vi "Data_select.vi"(6 "g(k) in 2":dbl[][](array[numeric]), 7 "s(k) Corregido":dbl[][](array[numeric]), 8 "m":i32=2, 9 "P":i32=64, 10 "s(k) in":dbl[][](array[numeric]), 11 "g(k) in":dbl[][](array[numeric])) -> (0 "s(k) lineal Corregido":ext[](array[numeric]), 1 "s(k) lineal":ext[](array[numeric]), 2 "g(k)lineal_2":ext[](array[numeric]), 3 "g(k) lineal":ext[](array[numeric]))   [LabVIEW 2015]
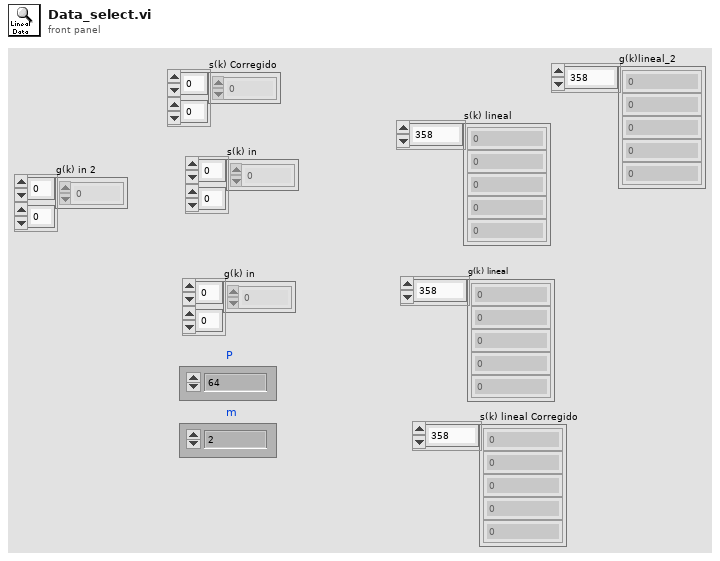
[diagram p1: front panel]
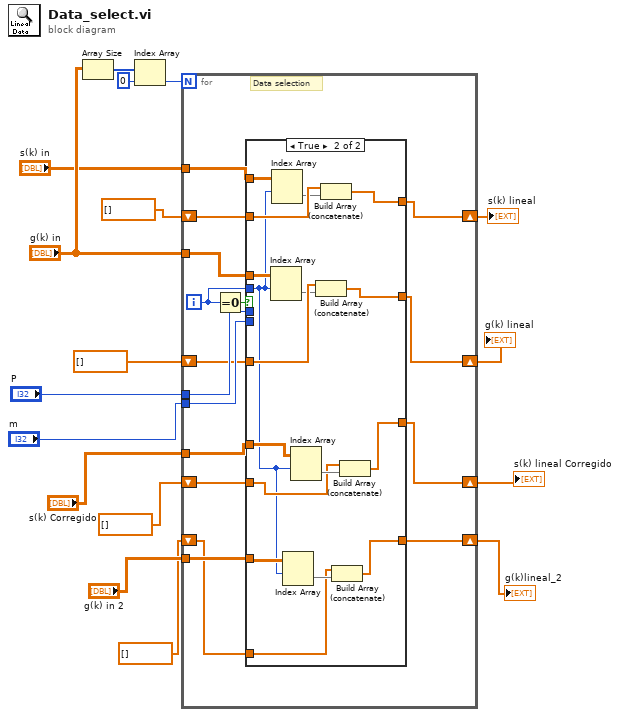
[diagram p0: block diagram]
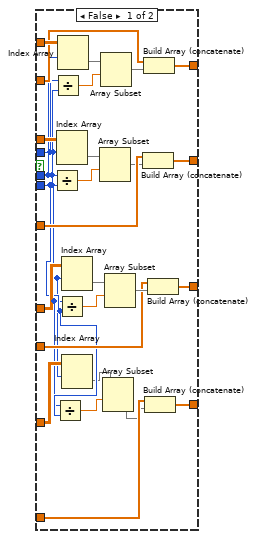
[diagram p2: hidden frame]
diagram:
  n1 = Array Size(array="g(k) in") -> (size(s)=w16:i32[])
  n2 = Index Array(array=w16, index=0) -> (element=w14:i32)
  n3 = for {
    N: w14 -> [_]
    tunnel: "g(k) in" -> [w32]
    tunnel: "m" -> [w30]
    tunnel: "P" -> [w29]
    shift-right: [w27] -> w10
    shift-left: ext[] [] ("Photon trace A") -> [w28]
    tunnel: "s(k) in" -> [w26]
    shift-right: [w24] -> w7
    shift-left: ext[] [] ("Photon trace A") -> [w25]
    tunnel: "s(k) Corregido" -> [w23]
    shift-right: [w21] -> w4
    shift-left: ext[] [] ("Photon trace A") -> [w22]
    tunnel: "g(k) in 2" -> [w20]
    shift-right: [w18] -> w1
    shift-left: ext[] [] ("Photon trace A") -> [w19]
    i -> [w31]
    # "Data selection"
    n4 = Equal To 0?(x=w31) -> (x = 0?=w33:bool)
    n5 = case shown="True" w33 {
      tunnel: w32 -> [w60 w77]
      tunnel: w31 -> [w38 w63]
      tunnel: w30 -> [w42 _]
      tunnel: w29 -> [w34 _]
      tunnel: w28 -> [w58 w76]
      tunnel: [w59 w74] -> w27
      tunnel: w26 -> [w51 w73]
      tunnel: w25 -> [w49 w72]
      tunnel: [w50 w70] -> w24
      tunnel: w23 -> [w45 w68]
      tunnel: w22 -> [w44 w67]
      tunnel: [w43 w66] -> w21
      tunnel: w20 -> [w39 w64]
      tunnel: w19 -> [w40 w62]
      tunnel: [w35 w61] -> w18
      frame False {
        n6 = Divide(x=w34, y=w42) -> (x/y=w56:dbl)
        n7 = Divide(x=w34, y=w42) -> (x/y=w53:dbl)
        n8 = Divide(x=w34, y=w42) -> (x/y=w41:dbl)
        n9 = Index Array(array=w60, index (row)=w38) -> (element=w57:dbl[])  [unwired: 1 in]
        n10 = Divide(x=w34, y=w42) -> (x/y=w47:dbl)
        n11 = Index Array(array=w51, index (row)=w38) -> (element=w54:dbl[])  [unwired: 1 in]
        n12 = Index Array(array=w45, index (row)=w38) -> (element=w48:dbl[])  [unwired: 1 in]
        n13 = Index Array(array=w39, index (row)=w38) -> (element=w37:dbl[])  [unwired: 1 in]
        n14 = Array Subset(array=w57, index=w56) -> (w55:dbl[])  [unwired: 1 in]
        n15 = Array Subset(array=w54, index=w53) -> (w52:dbl[])  [unwired: 1 in]
        n16 = Array Subset(array=w37, index=w41) -> (w36:dbl[])  [unwired: 1 in]
        n17 = Array Subset(array=w48, index=w47) -> (w46:dbl[])  [unwired: 1 in]
        n18 = Build Array (concatenate)(w58, w55) -> (w59:ext[])
        n19 = Build Array (concatenate)(w49, w52) -> (w50:ext[])
        n20 = Build Array (concatenate)(w40, w36) -> (w35:ext[])
        n21 = Build Array (concatenate)(w44, w46) -> (w43:ext[])
      }
      frame True {
        n22 = Index Array(array=w77, index (row)=w63) -> (element=w75:dbl[])  [unwired: 1 in]
        n23 = Index Array(array=w73, index (row)=w63) -> (element=w71:dbl[])  [unwired: 1 in]
        n24 = Index Array(array=w64, index (row)=w63) -> (element=w65:dbl[])  [unwired: 1 in]
        n25 = Index Array(array=w68, index (row)=w63) -> (element=w69:dbl[])  [unwired: 1 in]
        n26 = Build Array (concatenate)(w76, w75) -> (w74:ext[])
        n27 = Build Array (concatenate)(w72, w71) -> (w70:ext[])
        n28 = Build Array (concatenate)(w62, w65) -> (w61:ext[])
        n29 = Build Array (concatenate)(w67, w69) -> (w66:ext[])
      }
    }
  }
  "g(k) lineal" <- w10
  "s(k) lineal" <- w7
  "s(k) lineal Corregido" <- w4
  "g(k)lineal_2" <- w1
